vi "Main.vi"() -> ()   [LabVIEW 2024]
uses:
  C:/Users/ebarber/Documents/LabVIEW VIs/SolenoidGPT/autocom.dll
  autocom.dll
  <vilib>/JDP Science/JSONtext/JSONtext.lvlib
  e9269bf4-3461-4993-8ea8-2aebfbec4653.vi
  C:/Users/ebarber/Documents/LabVIEW VIs/SolenoidGPT/SpiController.dll
  SpiController.dll
  <vilib>/Instr/_visa.llb/VISA Configure Serial Port (Instr).vi
panel:
  out "concatenated string":string
  out "THIRD RESPONSE":string
  out "RESPONSE":string
  out "ECHO":string
  in  "VISA resource name":refnum<visa-resource-name>
  out "32 bit int out":string
  out "Command":string
  out "Parameters":dbl[](array[numeric])
  out "GetJLinkCOMPort":string
  in  "Please Select a Test":path
  in  "Run Test":bool
  in  "Configure Board":bool
  out "Board Connection Status":bool
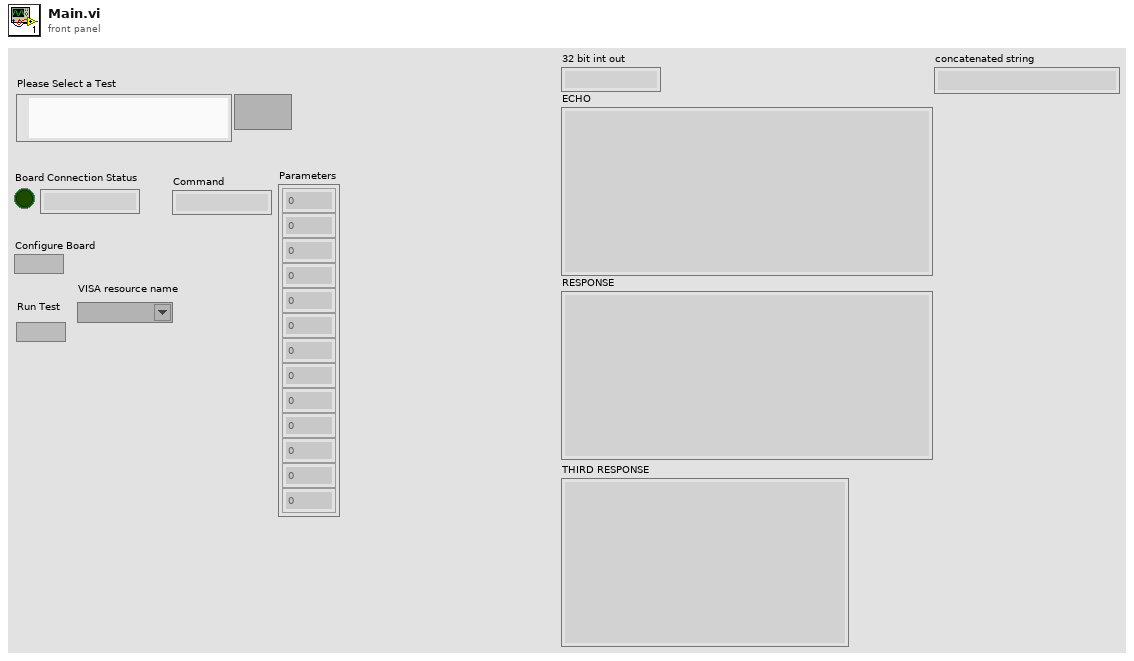
[diagram p1: front panel]
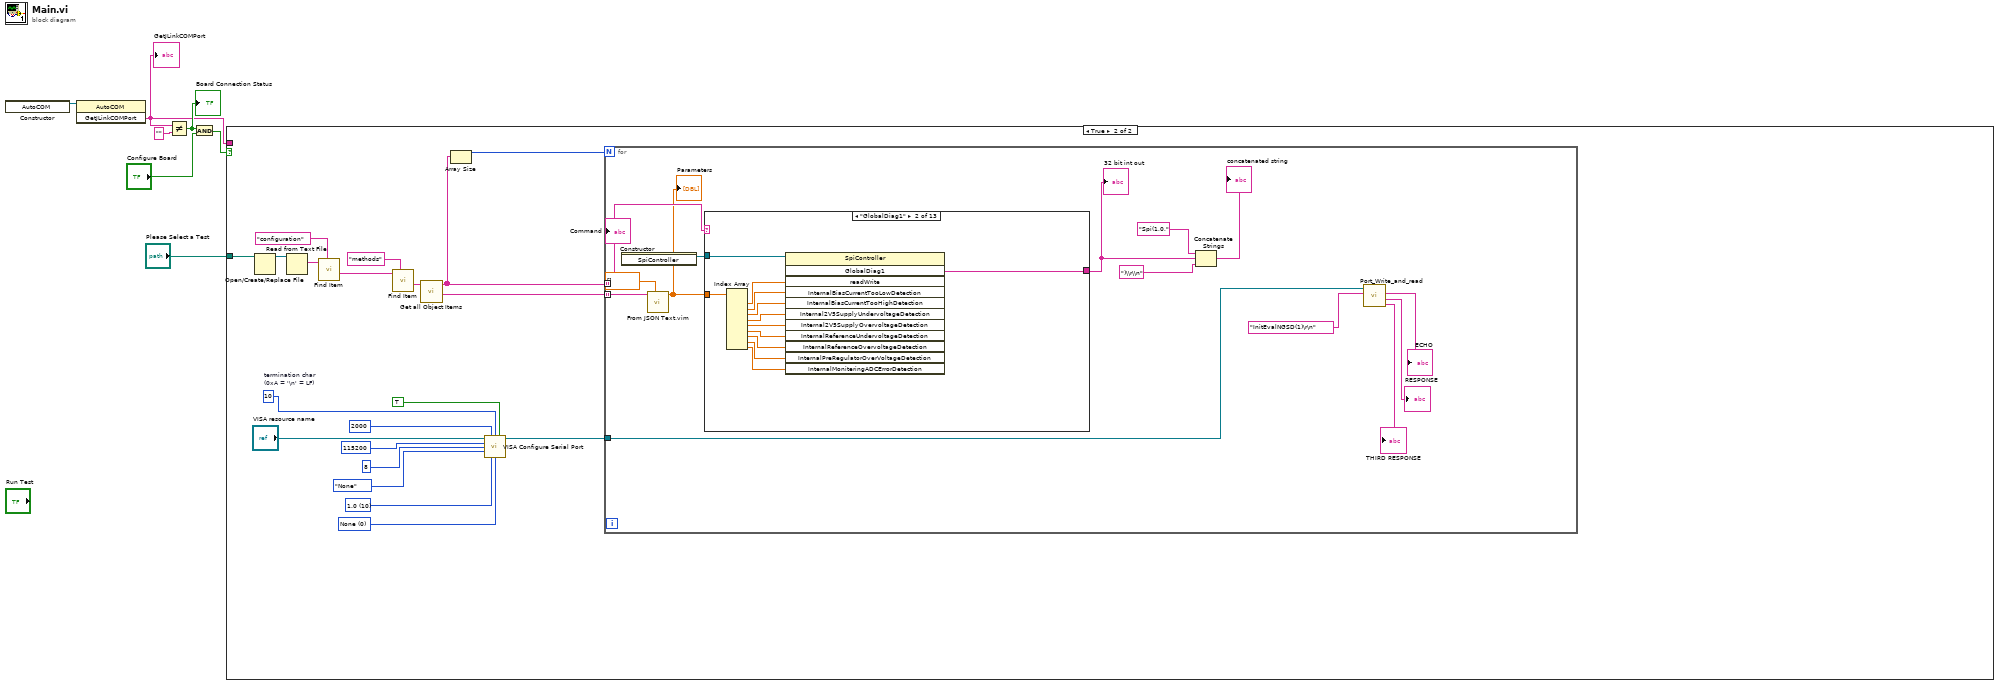
[diagram p0: block diagram]
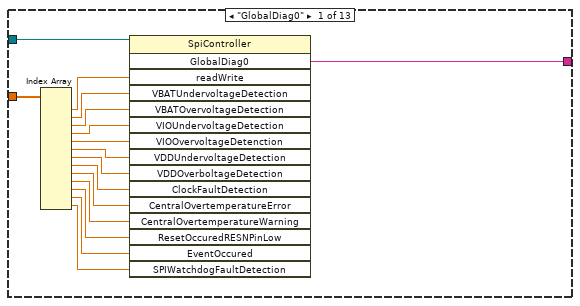
[diagram p3: hidden frame]
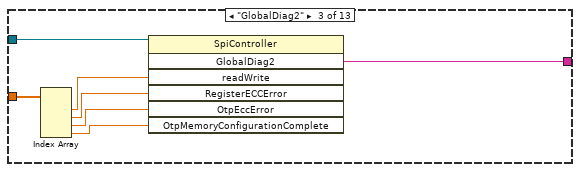
[diagram p4: hidden frame]
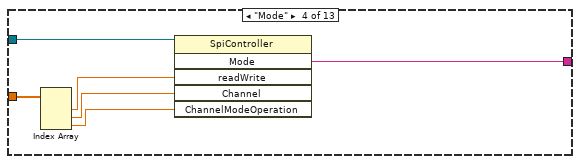
[diagram p5: hidden frame]
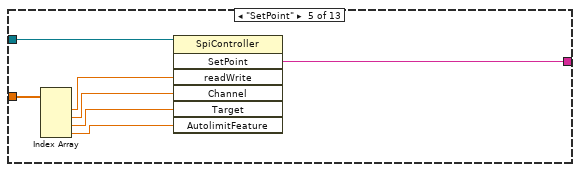
[diagram p6: hidden frame]
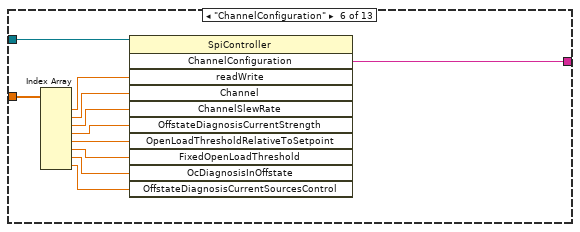
[diagram p7: hidden frame]
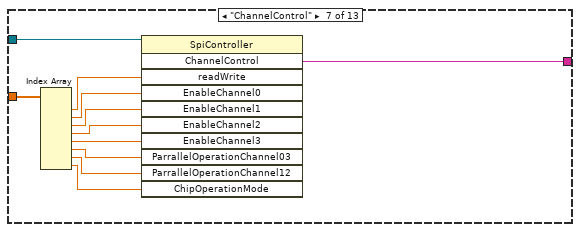
[diagram p8: hidden frame]
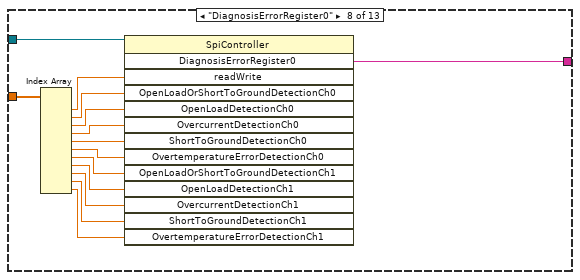
[diagram p9: hidden frame]
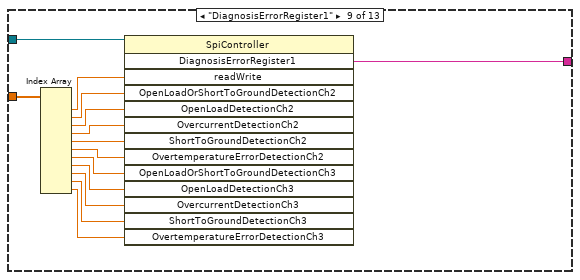
[diagram p10: hidden frame]
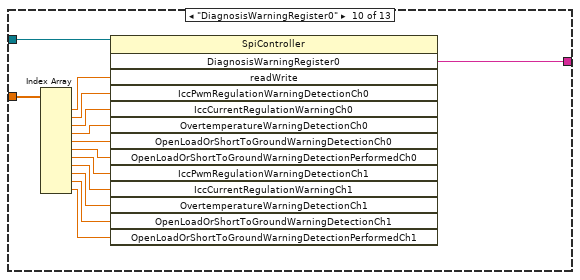
[diagram p11: hidden frame]
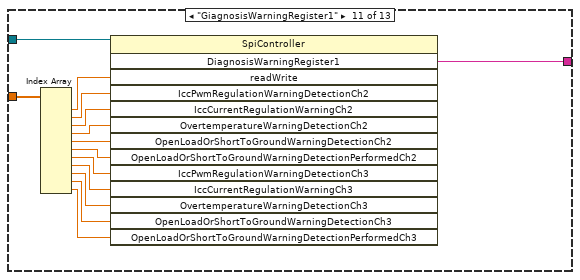
[diagram p12: hidden frame]
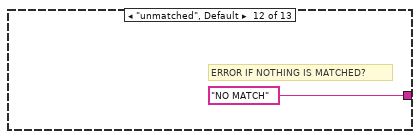
[diagram p13: hidden frame]
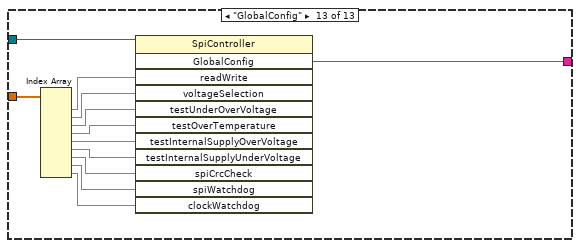
[diagram p14: hidden frame]
diagram:
  n1 = constructor class="AutoCOM"() -> (reference out=w7:refnum<k24>)  [unwired: 3 in, 2 out]
  n2 = invoke class="AutoCOM" method="GetJLinkCOMPort"(reference=w7) -> ("GetJLinkCOMPort"=w2:string)  [unwired: 2 in, 2 out]
  "GetJLinkCOMPort" <- w2
  n3 = Not Equal?(x=w2, y="") -> (x != y?=w4:bool)
  "Board Connection Status" <- w4
  n4 = And(x=w4, y="Configure Board") -> (x .and. y?=w5:bool)
  n5 = case shown="True" w5 {
    tunnel: w2 -> [_ _]
    tunnel: "Please Select a Test" -> [_ w27]
    frame False {
    }
    frame True {
      w9 = u16 0 items=["None", "XON/XOFF", "RTS/CTS", "XON/XOFF & RTS/CTS", "DTR/DSR", "XON/XOFF & DTR/DSR"] ("flow control (0:none)")
      w15 = u8 10  # termination char (0xA = '\n' = LF)
      w10 = u16 10 items=["1.0"=10, "1.5"=15, "2.0"=20] ("stop bits (10: 1 bit)")
      n6 = Open/Create/Replace File(file path (use dialog)=w27) -> (refnum out=w26:refnum<file>)  [unwired: 5 in, 2 out]
      n7 = Read from Text File(file (use dialog)=w26) -> (text=w25:string)  [unwired: 3 in, 3 out]
      n8 = call <vilib>:"Find Item.vi"("$Path or Item Name"="configuration", "JSON"=w25) -> ("<JSON>"=w23:string)  [unwired: 6 in, 3 out]
      n9 = call <vilib>:"Find Item.vi"("$Path or Item Name"="methods", "JSON"=w23) -> ("<JSON>"=w21:string)  [unwired: 6 in, 3 out]
      n10 = call <vilib>:"Get all Object Items.vi"("JSON"=w21) -> ("<JSON>"=w20:string[], "Item Names"=w19:string[])  [unwired: 7 in, 2 out]
      n11 = Array Size(array=w19) -> (size(s)=w18:i32)
      n12 = call-poly "VISA Configure Serial Port"("VISA resource name"="VISA resource name", "timeout (10sec)"=u32 2000, "termination char\n(0xA = '\\n' = LF)"=w15, "Enable Termination\nChar (T)"=TRUE ("Enable Termination\nChar (T)"), "baud rate (9600)"=u32 115200, "data bits (8)"=u16 8, "parity (0:none)"=enum16{"None", "Odd", "Even", "Mark", "Space"}."None", "stop bits (10: 1 bit)"=w10, "flow control (0:none)"=w9) -> ("VISA resource name out"=w8:refnum<visa-resource-name>)  [unwired: 5 in, 1 out]
      n13 = for {
        N: w18 -> [_]
        tunnel: w20 -> [w40] mode=indexing
        tunnel: w19 -> [w38] mode=indexing
        tunnel: w8 -> [w36]
        n14 = constructor class="SpiController"() -> (reference out=w39:refnum<k24>)  [unwired: 3 in, 2 out]
        n15 = call "From JSON Text.vim"("Data Type and Default Value"=dbl[] [], "JSON"=w40) -> ("Data out"=w37:dbl[])  [unwired: 8 in, 1 out]
        "Parameters" <- w37
        n16 = case shown="\"GlobalDiag1\"" w38 {
          tunnel: w39 -> [w57 w69 w76 w82 w89 w100 w111 w125 w139 w153 w167 _ w180]
          tunnel: [w56 w68 w75 w81 w88 w99 w110 w124 w138 w152 w166 "NO MATCH" w179] -> w34
          tunnel: w37 -> [w55 w67 w74 w80 w87 w98 w109 w123 w137 w151 w165 _ w178]
          frame "GlobalDiag0" {
            n17 = Index Array(array=w55) -> (element #1=w54:dbl, element #2=w53:dbl, element #3=w52:dbl, element #4=w51:dbl, element #5=w50:dbl, element #6=w49:dbl, element #7=w48:dbl, element #8=w47:dbl, element #9=w46:dbl, element #10=w45:dbl, element #11=w44:dbl, element #12=w43:dbl, element #13=w42:dbl)  [unwired: 13 in]
            n18 = invoke class="SpiController" method="GlobalDiag0"(reference=w57, "readWrite"=w54, "VBATUndervoltageDetection"=w53, "VBATOvervoltageDetection"=w52, "VIOUndervoltageDetection"=w51, "VIOOvervoltageDetenction"=w50, "VDDUndervoltageDetection"=w49, "VDDOverboltageDetection"=w48, "ClockFaultDetection"=w47, "CentralOvertemperatureError"=w46, "CentralOvertemperatureWarning"=w45, "ResetOccuredRESNPinLow"=w44, "EventOccured"=w43, "SPIWatchdogFaultDetection"=w42) -> ("GlobalDiag0"=w56:string)  [unwired: 2 in, 15 out]
          }
          frame "GlobalDiag1" {
            n19 = Index Array(array=w67) -> (element #1=w66:dbl, element #2=w65:dbl, element #3=w64:dbl, element #4=w63:dbl, element #5=w62:dbl, element #6=w61:dbl, element #7=w60:dbl, element #8=w59:dbl, element #9=w58:dbl)  [unwired: 9 in]
            n20 = invoke class="SpiController" method="GlobalDiag1"(reference=w69, "readWrite"=w66, "InternalBiasCurrentTooLowDetection"=w65, "InternalBiasCurrentTooHighDetection"=w64, "Internal2V5SupplyUndervoltageDetection"=w63, "Internal2V5SupplyOvervoltageDetection"=w62, "InternalReferenceUndervoltageDetection"=w61, "InternalReferenceOvervoltageDetection"=w60, "InternalPreRegulatorOverVoltageDetection"=w59, "InternalMoniteringADCErrorDetection"=w58) -> ("GlobalDiag1"=w68:string)  [unwired: 2 in, 11 out]
          }
          frame "GlobalDiag2" {
            n21 = Index Array(array=w74) -> (element #1=w73:dbl, element #2=w72:dbl, element #3=w71:dbl, element #4=w70:dbl)  [unwired: 4 in]
            n22 = invoke class="SpiController" method="GlobalDiag2"(reference=w76, "readWrite"=w73, "RegisterECCError"=w72, "OtpEccError"=w71, "OtpMemoryConfigurationComplete"=w70) -> ("GlobalDiag2"=w75:string)  [unwired: 2 in, 6 out]
          }
          frame "Mode" {
            n23 = Index Array(array=w80) -> (element #1=w79:dbl, element #2=w78:dbl, element #3=w77:dbl)  [unwired: 3 in]
            n24 = invoke class="SpiController" method="Mode"(reference=w82, "readWrite"=w79, "Channel"=w78, "ChannelModeOperation"=w77) -> ("Mode"=w81:string)  [unwired: 2 in, 5 out]
          }
          frame "SetPoint" {
            n25 = Index Array(array=w87) -> (element #1=w86:dbl, element #2=w85:dbl, element #3=w84:dbl, element #4=w83:dbl)  [unwired: 4 in]
            n26 = invoke class="SpiController" method="SetPoint"(reference=w89, "readWrite"=w86, "Channel"=w85, "Target"=w84, "AutolimitFeature"=w83) -> ("SetPoint"=w88:string)  [unwired: 2 in, 6 out]
          }
          frame "ChannelConfiguration" {
            n27 = Index Array(array=w98) -> (element #1=w97:dbl, element #2=w96:dbl, element #3=w95:dbl, element #4=w94:dbl, element #5=w93:dbl, element #6=w92:dbl, element #7=w91:dbl, element #8=w90:dbl)  [unwired: 8 in]
            n28 = invoke class="SpiController" method="ChannelConfiguration"(reference=w100, "readWrite"=w97, "Channel"=w96, "ChannelSlewRate"=w95, "OffstateDiagnosisCurrentStrength"=w94, "OpenLoadThresholdRelativeToSetpoint"=w93, "FixedOpenLoadThreshold"=w92, "OcDiagnosisInOffstate"=w91, "OffstateDiagnosisCurrentSourcesControl"=w90) -> ("ChannelConfiguration"=w99:string)  [unwired: 2 in, 10 out]
          }
          frame "ChannelControl" {
            n29 = Index Array(array=w109) -> (element #1=w108:dbl, element #2=w101:dbl, element #3=w107:dbl, element #4=w106:dbl, element #5=w105:dbl, element #6=w104:dbl, element #7=w103:dbl, element #8=w102:dbl)  [unwired: 8 in]
            n30 = invoke class="SpiController" method="ChannelControl"(reference=w111, "readWrite"=w108, "EnableChannel0"=w101, "EnableChannel1"=w107, "EnableChannel2"=w106, "EnableChannel3"=w105, "ParrallelOperationChannel03"=w104, "ParrallelOperationChannel12"=w103, "ChipOperationMode"=w102) -> ("ChannelControl"=w110:string)  [unwired: 2 in, 10 out]
          }
          frame "DiagnosisErrorRegister0" {
            n31 = Index Array(array=w123) -> (element #1=w122:dbl, element #2=w121:dbl, element #3=w120:dbl, element #4=w119:dbl, element #5=w118:dbl, element #6=w117:dbl, element #7=w116:dbl, element #8=w115:dbl, element #9=w114:dbl, element #10=w113:dbl, element #11=w112:dbl)  [unwired: 11 in]
            n32 = invoke class="SpiController" method="DiagnosisErrorRegister0"(reference=w125, "readWrite"=w122, "OpenLoadOrShortToGroundDetectionCh0"=w121, "OpenLoadDetectionCh0"=w120, "OvercurrentDetectionCh0"=w119, "ShortToGroundDetectionCh0"=w118, "OvertemperatureErrorDetectionCh0"=w117, "OpenLoadOrShortToGroundDetectionCh1"=w116, "OpenLoadDetectionCh1"=w115, "OvercurrentDetectionCh1"=w114, "ShortToGroundDetectionCh1"=w113, "OvertemperatureErrorDetectionCh1"=w112) -> ("DiagnosisErrorRegister0"=w124:string)  [unwired: 2 in, 13 out]
          }
          frame "DiagnosisErrorRegister1" {
            n33 = Index Array(array=w137) -> (element #1=w136:dbl, element #2=w135:dbl, element #3=w134:dbl, element #4=w133:dbl, element #5=w132:dbl, element #6=w131:dbl, element #7=w130:dbl, element #8=w129:dbl, element #9=w128:dbl, element #10=w127:dbl, element #11=w126:dbl)  [unwired: 11 in]
            n34 = invoke class="SpiController" method="DiagnosisErrorRegister1"(reference=w139, "readWrite"=w136, "OpenLoadOrShortToGroundDetectionCh2"=w135, "OpenLoadDetectionCh2"=w134, "OvercurrentDetectionCh2"=w133, "ShortToGroundDetectionCh2"=w132, "OvertemperatureErrorDetectionCh2"=w131, "OpenLoadOrShortToGroundDetectionCh3"=w130, "OpenLoadDetectionCh3"=w129, "OvercurrentDetectionCh3"=w128, "ShortToGroundDetectionCh3"=w127, "OvertemperatureErrorDetectionCh3"=w126) -> ("DiagnosisErrorRegister1"=w138:string)  [unwired: 2 in, 13 out]
          }
          frame "DiagnosisWarningRegister0" {
            n35 = Index Array(array=w151) -> (element #1=w150:dbl, element #2=w149:dbl, element #3=w148:dbl, element #4=w147:dbl, element #5=w146:dbl, element #6=w145:dbl, element #7=w144:dbl, element #8=w143:dbl, element #9=w142:dbl, element #10=w141:dbl, element #11=w140:dbl)  [unwired: 11 in]
            n36 = invoke class="SpiController" method="DiagnosisWarningRegister0"(reference=w153, "readWrite"=w150, "IccPwmRegulationWarningDetectionCh0"=w149, "IccCurrentRegulationWarningCh0"=w148, "OvertemperatureWarningDetectionCh0"=w147, "OpenLoadOrShortToGroundWarningDetectionCh0"=w146, "OpenLoadOrShortToGroundWarningDetectionPerformedCh0"=w145, "IccPwmRegulationWarningDetectionCh1"=w144, "IccCurrentRegulationWarningCh1"=w143, "OvertemperatureWarningDetectionCh1"=w142, "OpenLoadOrShortToGroundWarningDetectionCh1"=w141, "OpenLoadOrShortToGroundWarningDetectionPerformedCh1"=w140) -> ("DiagnosisWarningRegister0"=w152:string)  [unwired: 2 in, 13 out]
          }
          frame "GiagnosisWarningRegister1" {
            n37 = Index Array(array=w165) -> (element #1=w164:dbl, element #2=w163:dbl, element #3=w162:dbl, element #4=w161:dbl, element #5=w160:dbl, element #6=w159:dbl, element #7=w158:dbl, element #8=w157:dbl, element #9=w156:dbl, element #10=w155:dbl, element #11=w154:dbl)  [unwired: 11 in]
            n38 = invoke class="SpiController" method="DiagnosisWarningRegister1"(reference=w167, "readWrite"=w164, "IccPwmRegulationWarningDetectionCh2"=w163, "IccCurrentRegulationWarningCh2"=w162, "OvertemperatureWarningDetectionCh2"=w161, "OpenLoadOrShortToGroundWarningDetectionCh2"=w160, "OpenLoadOrShortToGroundWarningDetectionPerformedCh2"=w159, "IccPwmRegulationWarningDetectionCh3"=w158, "IccCurrentRegulationWarningCh3"=w157, "OvertemperatureWarningDetectionCh3"=w156, "OpenLoadOrShortToGroundWarningDetectionCh3"=w155, "OpenLoadOrShortToGroundWarningDetectionPerformedCh3"=w154) -> ("DiagnosisWarningRegister1"=w166:string)  [unwired: 2 in, 13 out]
          }
          frame "unmatched", Default {
            # "ERROR IF NOTHING IS MATCHED?"
          }
          frame "GlobalConfig" {
            n39 = Index Array(array=w178) -> (element #1=w177:dbl, element #2=w176:dbl, element #3=w175:dbl, element #4=w174:dbl, element #5=w173:dbl, element #6=w172:dbl, element #7=w171:dbl, element #8=w170:dbl, element #9=w169:dbl)  [unwired: 9 in]
            n40 = invoke class="SpiController" method="GlobalConfig"(reference=w180, "readWrite"=w177, "voltageSelection"=w176, "testUnderOverVoltage"=w175, "testOverTemperature"=w174, "testInternalSupplyOverVoltage"=w173, "testInternalSupplyUnderVoltage"=w172, "spiCrcCheck"=w171, "spiWatchdog"=w170, "clockWatchdog"=w169) -> ("GlobalConfig"=w179:string)  [unwired: 2 in, 11 out]
          }
        }
        "32 bit int out" <- w34
        n41 = Concatenate Strings("Spi(1,0," ("string"), w34, ")\\r\\n" ("string")) -> (→"concatenated string":string)
        n42 = call "Port_Write_and_read.vi"("write buffer"="InitEvalNGSD(1)\r\n", "VISA Refnum in"=w36) -> ("read buffer"=→"THIRD RESPONSE":string, "read buffer 2"=→"RESPONSE":string, "read buffer 3"=→"ECHO":string)  [unwired: 4 in, 1 out]
        "Command" <- w38
      }
    }
  }
